vi "Register gRPC Methods.vi"(8 "error in (no error)":errorcluster, 11 "gRPC service in":refnum<class "streamai.lvclass">) -> (0 "error out":errorcluster, 3 "gRPC service out":refnum<class "streamai.lvclass">)   [LabVIEW 2023, in "Generated_server.lvlib" / "streamai.lvclass"]
uses:
  streamai.lvclass
  typeDefs/Server Internal UEs.ctl
  typeDefs/Server Internal Message.ctl
  typeDefs/Server gRPC UEs.ctl
  <vilib>/gRPC/LabVIEW gRPC Library/Server API/typeDefs/gRPCId Cluster.ctl
  <vilib>/gRPC/LabVIEW gRPC Library/Shared/grpcId.ctl
  streamai.lvclass/streamai.ctl
  <vilib>/gRPC/LabVIEW gRPC Library/grpc-lvsupport-release.lvlib
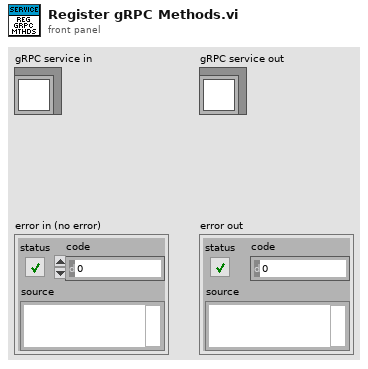
[diagram p1: front panel]
types:
  T1 = typedef "Generated_server.lvlib/streamai.lvclass/Server gRPC UEs.ctl" = cluster{"streamai startacq gRPC UE":refnum<user-event>, "streamai stopacq gRPC UE":refnum<user-event>, "streamai setSignalConfig gRPC UE":refnum<user-event>, "streamai setSamplingConfig gRPC UE":refnum<user-event>}
  T2 = typedef "Generated_server.lvlib/streamai.lvclass/Server Internal UEs.ctl" = cluster{"streamai startacq Internal UE":refnum<user-event>, "streamai stopacq Internal UE":refnum<user-event>, "streamai setSignalConfig Internal UE":refnum<user-event>, "streamai setSamplingConfig Internal UE":refnum<user-event>}
  T3 = typedef "grpc-lvsupport-release.lvlib/grpcId.ctl" = u64
  T4 = typedef "Generated_server.lvlib/streamai.lvclass/Server Internal Message UE.ctl" = refnum<user-event>
  T5 = typedef "grpc-lvsupport-release.lvlib/gRPCId Cluster UE.ctl" = refnum<user-event>
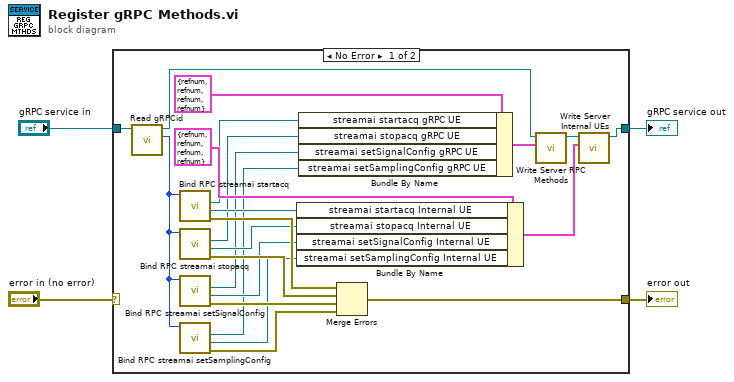
[diagram p0: block diagram]
diagram:
  n1 = case shown="No Error" "error in (no error)" {
    selector: "error in (no error)" -> [_ w27]
    tunnel: "gRPC service in" -> [w18 w28]
    tunnel: [w26 w27] -> w3
    tunnel: [w25 w28] -> w2
    frame No Error {
      n2 = call-dynamic "Read gRPCid.vi"("gRPC service in"=w18) -> ("gRPCid"=w17:T3, "gRPC service out"=w19:refnum<class "streamai.lvclass">)  [unwired: 8 in, 1 out]
      n3 = call "Bind RPC streamai startacq.vi"("gRPCid server in"=w17) -> ("error out"=w16:errorcluster, "streamai startacq Internal UE"=w14:T4, "streamai startacq gRPC UE"=w15:T5)  [unwired: 7 in, 1 out]
      n4 = call "Bind RPC streamai stopacq.vi"("gRPCid server in"=w17) -> ("error out"=w13:errorcluster, "streamai stopacq Internal UE"=w11:T4, "streamai stopacq gRPC UE"=w12:T5)  [unwired: 7 in, 1 out]
      n5 = call "Bind RPC streamai setSignalConfig.vi"("gRPCid server in"=w17) -> ("error out"=w10:errorcluster, "streamai setSignalConfig Internal UE"=w8:T4, "streamai setSignalConfig gRPC UE"=w9:T5)  [unwired: 7 in, 1 out]
      n6 = call "Bind RPC streamai setSamplingConfig.vi"("gRPCid server in"=w17) -> ("error out"=w7:errorcluster, "streamai setSamplingConfig Internal UE"=w5:T4, "streamai setSamplingConfig gRPC UE"=w6:T5)  [unwired: 7 in, 1 out]
      n7 = Bundle By Name ("Bundle Internal UEs")(cluster=T2 {"streamai startacq Internal UE"=refnum, "streamai stopacq Internal UE"=refnum, "streamai setSignalConfig Internal UE"=refnum, "streamai setSamplingConfig Internal UE"=refnum} ("Server Internal UEs"), "streamai startacq Internal UE"=w14, "streamai stopacq Internal UE"=w11, "streamai setSignalConfig Internal UE"=w8, "streamai setSamplingConfig Internal UE"=w5) -> (w24:T2)
      n8 = Bundle By Name ("Bundle gRPC UEs")(cluster=T1 {"streamai startacq gRPC UE"=refnum, "streamai stopacq gRPC UE"=refnum, "streamai setSignalConfig gRPC UE"=refnum, "streamai setSamplingConfig gRPC UE"=refnum} ("gRPC Server Method Events"), "streamai startacq gRPC UE"=w15, "streamai stopacq gRPC UE"=w12, "streamai setSignalConfig gRPC UE"=w9, "streamai setSamplingConfig gRPC UE"=w6) -> (w21:T1)
      n9 = Merge Errors(w16, w13, w10, w7) -> (w26:errorcluster)
      n10 = call "Write Server RPC Methods.vi"("Server RPC Methods"=w21, "gRPC service in"=w19) -> ("gRPC service out"=w22:refnum<class "streamai.lvclass">)  [unwired: 8 in, 1 out]
      n11 = call "Write Server Internal UEs.vi"("Server Internal UEs"=w24, "gRPC service in"=w22) -> ("gRPC service out"=w25:refnum<class "streamai.lvclass">)  [unwired: 8 in, 1 out]
    }
    frame Error {
    }
  }
  "error out" <- w3
  "gRPC service out" <- w2
